vi "Configure Ripple Limit Test.vi"(5 "Display Type (0: Off)":i32(ring) items=["Off", "Absolute", "Margin"], 6 "Limit Band Value (1)":i32=1, 7 "Enable Ripple Limit Test (F: Disable)":bool, 8 "error in (no error)":errorcluster, 9 "Enable Ripple Limit Line Display (T: Enable)":bool=TRUE, 10 "Channel (1)":i32=1, 11 "VISA resource name":refnum<visa-resource-name>) -> (0 "error out":errorcluster, 3 "VISA resource name out":refnum<visa-resource-name>)   [LabVIEW 2022 SP3, in "Agilent ENA Series.lvlib"]
doc: "Configures the ripple limit test."
uses:
  <instrlib>/Agilent ENA Series/Agilent ENA Series.lvlib
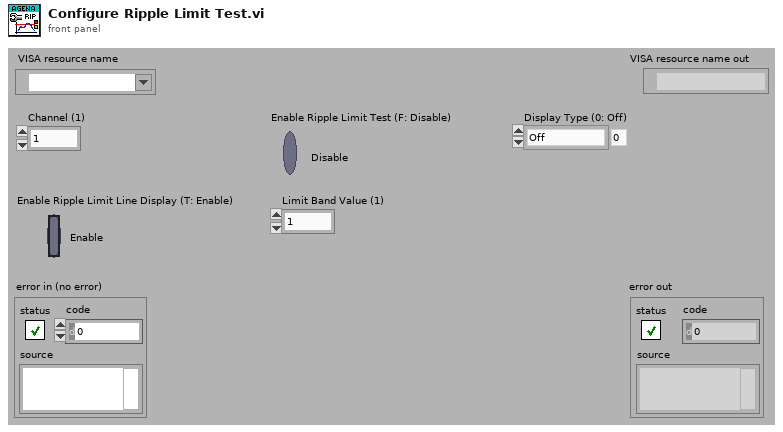
[diagram p1: front panel]
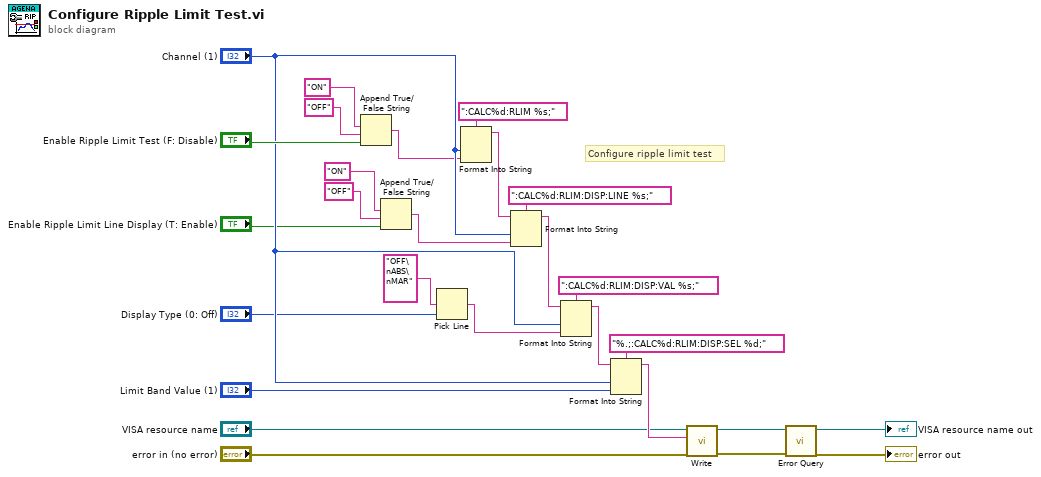
[diagram p0: block diagram]
diagram:
  # "Configure ripple limit test"
  n1 = Append True/False String(1:"Enable Ripple Limit Test (F: Disable)", 2:"OFF", 3:"ON") -> (0:w22:string)  [unwired: 1 out]
  n2 = Append True/False String(1:"Enable Ripple Limit Line Display (T: Enable)", 2:"OFF", 3:"ON") -> (0:w16:string)  [unwired: 1 out]
  n3 = Pick Line(multi-line string="OFF\nABS\nMAR", line index="Display Type (0: Off)") -> (output string=w11:string)  [unwired: 1 out]
  n4 = Format Into String(format string=":CALC%d:RLIM %s;", "Channel (1)", w22) -> (resulting string=w18:string)  [unwired: 2 in, 1 out]
  n5 = Format Into String(format string=":CALC%d:RLIM:DISP:LINE %s;", initial string=w18, "Channel (1)", w16) -> (resulting string=w13:string)  [unwired: 1 in, 1 out]
  n6 = Format Into String(format string=":CALC%d:RLIM:DISP:VAL %s;", initial string=w13, "Channel (1)", w11) -> (resulting string=w10:string)  [unwired: 1 in, 1 out]
  n7 = Format Into String(format string="%.;:CALC%d:RLIM:DISP:SEL %d;", initial string=w10, "Channel (1)", "Limit Band Value (1)") -> (resulting string=w3:string)  [unwired: 1 in, 1 out]
  n8 = call <instrlib>:"Write.vi"("error in (no error)"="error in (no error)", "String ()"=w3, "VISA resource name"="VISA resource name") -> ("error out"=w4:errorcluster, "VISA resource name out"=w5:refnum<visa-resource-name>)  [unwired: 6 in, 1 out]
  n9 = call <instrlib>:"Error Query.vi"("error in (no error)"=w4, "VISA resource name"=w5) -> ("error out"=→"error out":errorcluster, "VISA resource name out"=→"VISA resource name out":refnum<visa-resource-name>)  [unwired: 8 out]
